vi "生成CODMn data (子VI).vi"() -> (3 "data":T1)   [LabVIEW 2016]
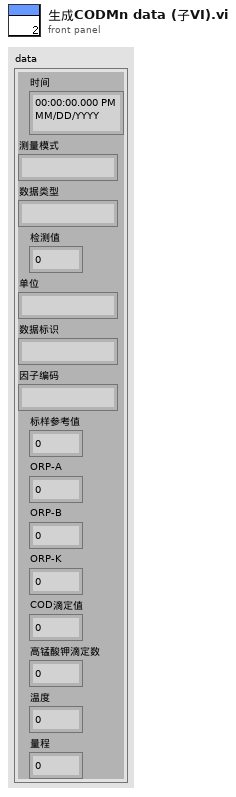
[diagram p1: front panel]
types:
  T1 = cluster{"时间":timestamp, "测量模式":string, "数据类型":string, "检测值":sgl, "单位":string, "数据标识":string, "因子编码":string, "标样参考值":sgl, "ORP-A":sgl, "ORP-B":sgl, "ORP-K":sgl, "COD滴定值":sgl, "高锰酸钾滴定数":sgl, "温度":sgl, "量程":sgl}
  T2 = cluster{"运行模式":enum16{"维护模式", "常规模式", "应急模式", "质控模式"}}
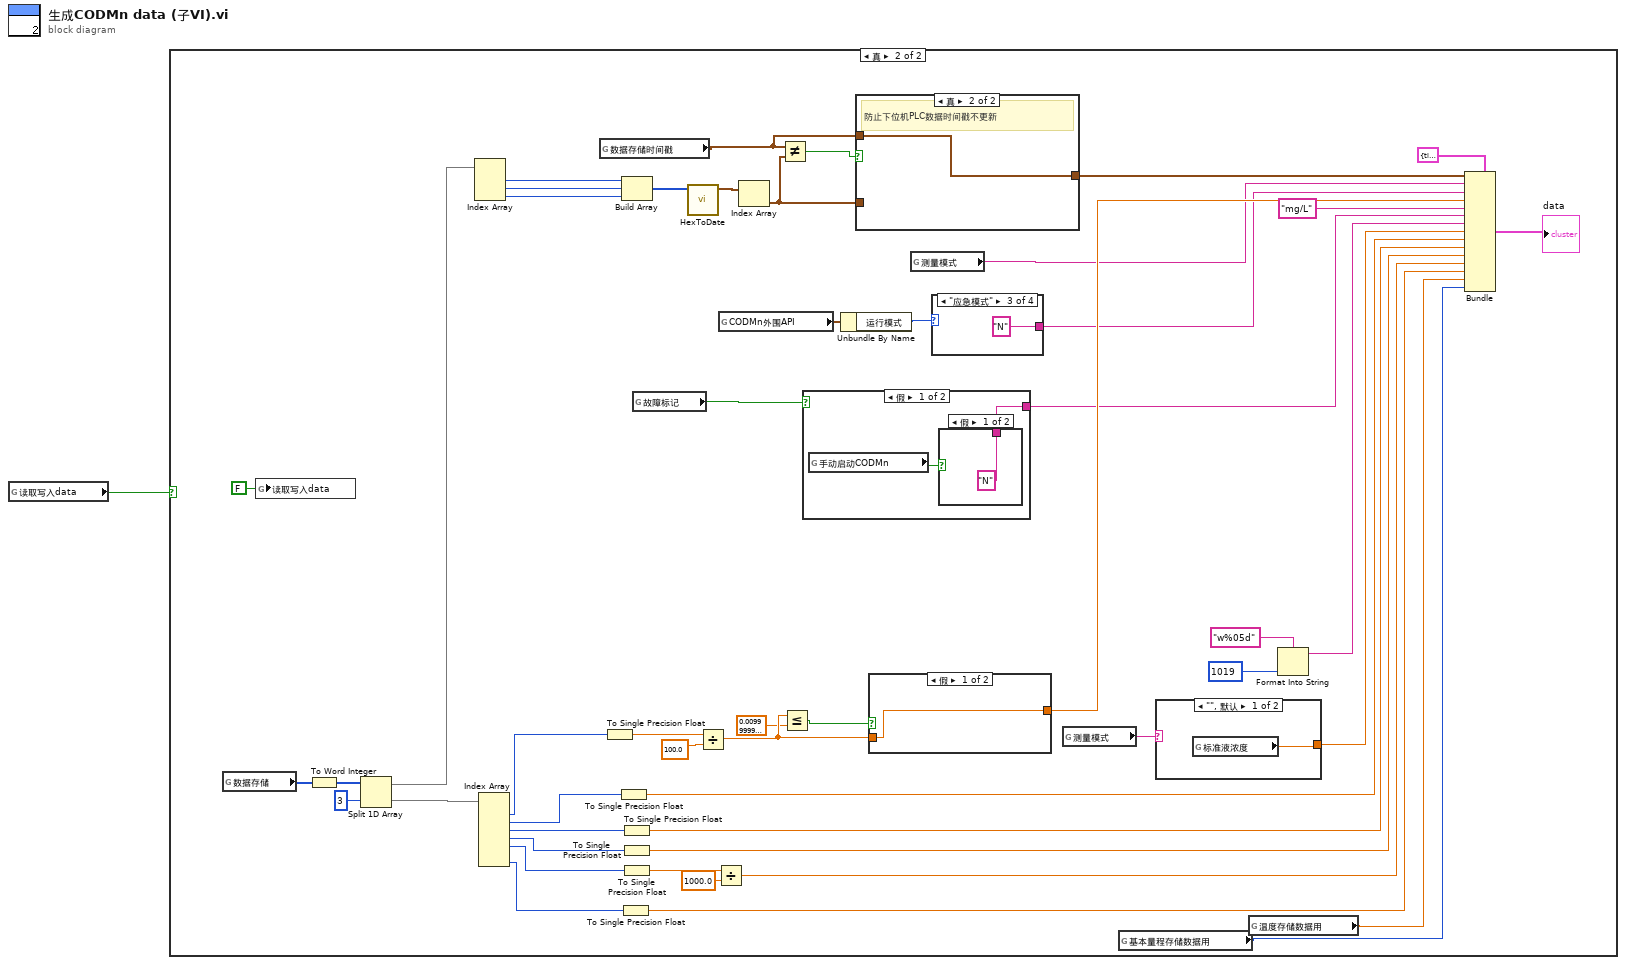
[diagram p0: block diagram]
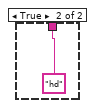
[diagram p4: hidden frame]
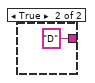
[diagram p5: hidden frame]
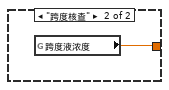
[diagram p6: hidden frame]
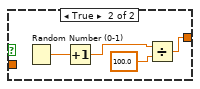
[diagram p7: hidden frame]
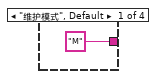
[diagram p8: hidden frame]
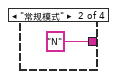
[diagram p9: hidden frame]
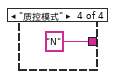
[diagram p10: hidden frame]
diagram:
  n1 = global read "COD读取DATA全局.vi" "读取写入data"() -> (w1:bool)
  n2 = case shown="真" w1 {
    frame False {
    }
    frame True {
      n3 = global read "COD读取DATA全局.vi" "数据存储"() -> (w46:u16[])
      n4 = global write "COD读取DATA全局.vi" "读取写入data"(FALSE ("读取写入data")) -> ()
      n5 = To Word Integer(number=w46) -> (16bit integer=w35:i16[])
      n6 = Split 1D Array(array=w35, index=3 ("索引")) -> (first subarray=w5:i16[], second subarray=w15:i16[])
      n7 = Index Array(array=w5) -> (element #1=w7:i16, element #2=w8:i16, element #3=w9:i16)  [unwired: 3 in]
      n8 = Index Array(array=w15) -> (element #1=w34:i16, element #2=w11:i16, element #3=w12:i16, element #4=w13:i16, element #5=w14:i16, element #7=w48:i16)  [unwired: 7 in, 1 out]
      n9 = global read "COD读取DATA全局.vi" "数据存储时间戳"() -> (w49:timestamp)
      n10 = To Single Precision Float(number=w34) -> (single precision float=w32:sgl)
      n11 = To Single Precision Float(number=w11) -> (single precision float=w24:sgl)
      n12 = To Single Precision Float(number=w48) -> (single precision float=w29:sgl)
      n13 = Build Array(w7, w8, w9) -> (w10:i16[])
      n14 = To Single Precision Float(number=w12) -> (single precision float=w23:sgl)
      n15 = To Single Precision Float(number=w13) -> (single precision float=w22:sgl)
      n16 = To Single Precision Float(number=w14) -> (single precision float=w18:sgl)
      n17 = global read "COD读取DATA全局.vi" "故障标记"() -> (w51:bool)
      n18 = call "HexToDate.vi"("数组"=w10) -> ("DATE"=w6:timestamp[])  [unwired: 10 in]
      n19 = Divide(x=w32, y=sgl 100.0) -> (x/y=w33:sgl)
      n20 = Divide(x=w18, y=sgl 1000.0) -> (x/y=w21:sgl)
      n21 = global read "CODMN外部API.vi" "CODMn外围API"() -> (w40:T2)
      n22 = Index Array(array=w6) -> (element=w43:timestamp)  [unwired: 1 in]
      n23 = Not Equal?(x=w49, y=w43) -> (x != y?=w44:bool)
      n24 = Less Or Equal?(x=w33, y=sgl 0.01) -> (x <= y?=w31:bool)
      n25 = case shown="假" w51 {
        tunnel: [w55 "D" ("数据标识")] -> w26
        frame False {
          n26 = global read "CODMN外部API.vi" "手动启动CODMn"() -> (w54:bool)
          n27 = case shown="假" w54 {
            tunnel: ["N" ("数据标识") "hd" ("数据标识")] -> w55
            frame False {
            }
            frame True {
            }
          }
        }
        frame True {
        }
      }
      n28 = Unbundle By Name(w40) -> ("运行模式"=w41:enum16{"维护模式", "常规模式", "应急模式", "质控模式"})
      n29 = case "条件结构" shown="真" w44 {
        tunnel: w43 -> [w52 _]
        tunnel: w49 -> [_ w53]
        tunnel: [w52 w53] -> w45
        frame False {
        }
        frame True {
          # "防止下位机PLC数据时间戳不更新"
        }
      }
      n30 = case shown="假" w31 {
        tunnel: [w61 w62] -> w47
        tunnel: w33 -> [w61 _]
        frame False {
        }
        frame True {
          n31 = Random Number (0-1)() -> (number: 0 to 1=w65:dbl)
          n32 = Increment(x=w65) -> (x+1=w63:dbl)
          n33 = Divide(x=w63, y=sgl 100.0) -> (x/y=w62:dbl)
        }
      }
      n34 = global read "COD测量模式全局.vi" "测量模式"() -> (w42:string)
      n35 = case shown="\"应急模式\"" w41 {
        tunnel: ["M" ("单位") "N" ("单位") "N" ("单位") "N" ("单位")] -> w28
        frame "维护模式", Default {
        }
        frame "常规模式" {
        }
        frame "应急模式" {
        }
        frame "质控模式" {
        }
      }
      n36 = global read "COD测量模式全局.vi" "测量模式"() -> (w36:string)
      n37 = global read "COD读取DATA全局.vi" "基本量程存储数据用"() -> (w3:enum16{"L", "H"})
      n38 = case shown="\"\", 默认" w36 {
        tunnel: [w59 w60] -> w37
        frame "", Default {
          n39 = global read "COD浓度全局变量.vi" "标准液浓度"() -> (w59:dbl)
        }
        frame "跨度核查" {
          n40 = global read "CODMn断电保存全局变量.vi" "跨度液浓度"() -> (w60:dbl)
        }
      }
      n41 = global read "COD读取DATA全局.vi" "温度存储数据用"() -> (w50:dbl)
      n42 = Format Into String(format string="w%05d" ("格式字符串"), u32 1019 ("因子编码")) -> (resulting string=w25:string)  [unwired: 2 in, 1 out]
      n43 = Bundle(cluster=T1 {"时间"=timestamp(0 s since 1904-01-01), "测量模式"="", "数据类型"="", "检测值"=0.0, "单位"="", "数据标识"="", "因子编码"="", "标样参考值"=0.0, "ORP-A"=0.0, "ORP-B"=0.0, "ORP-K"=0.0, "COD滴定值"=0.0, "高锰酸钾滴定数"=0.0, "温度"=0.0, "量程"=0.0} ("data"), "时间"=w45, "测量模式"=w42, "数据类型"=w28, "检测值"=w47, "单位"="mg/L", "数据标识"=w26, "因子编码"=w25, "标样参考值"=w37, "ORP-A"=w24, "ORP-B"=w23, "ORP-K"=w22, "COD滴定值"=w21, "高锰酸钾滴定数"=w29, "温度"=w50, "量程"=w3) -> (→"data":T1)
    }
  }
